vi "user status.vi"(0 "User Index in":i32, 2 "User Info":refnum<vi>, 7 "Userdatabase":path=path "C:/Program Files/National Instruments/LabVIEW 8.2/userdatabase", 9 "User Options":refnum<vi>, 11 "error in (no error)":errorcluster, 12 "User status cmd":T3=enum."Load inputs") -> (3 "valid form":bool, 4 "User Index":i32, 6 "User Information out":T1 {"Country" items=["Afghanistan", "Aland Islands", "Albania", "Algeria", "American Samoa", "Andorra", "Angola", "Anguilla", "Antarctica", "Antigua And Barbuda", "Argentina", "Armenia", "Aruba", "Australia", "Austria", "Azerbaijan", "Bahamas", "Bahrain", "Bangladesh", "Barbados", "Belarus", "Belgium", "Belize", "Benin", "Bermuda", "Bhutan", "Bolivia", "Bosnia And Herzegovina", "Botswana", "Bouvet Island", "Brazil", "British Indian Ocean Territory", "Brunei Darussalam", "Bulgaria", "Burkina Faso", "Burundi", "Cambodia", "Cameroon", "Canada", "Cape Verde", "Cayman Islands", "Central African Republic", "Chad", "Chile", "China", "Christmas Island", "Cocos (Keeling) Islands", "Colombia", "Comoros", "Congo", "Congo, The Democratic Republic Of The", "Cook Islands", "Costa Rica", "Cote D'Ivoire", "Croatia", "Cuba", "Cyprus", "Czech Republic", "Denmark", "Djibouti", "Dominica", "Dominican Republic", "Ecuador", "Egypt", "El Salvador", "Equatorial Guinea", "Eritrea", "Estonia", "Ethiopia", "Falkland Islands (Malvinas)", "Faroe Islands", "Fiji", "Finland", "France", "French Guiana", "French Polynesia", "French Southern Territories", "Gabon", "Gambia", "Georgia", "Germany", "Ghana", "Gibraltar", "Greece", "Greenland", "Grenada", "Guadeloupe", "Guam", "Guatemala", "Guernsey", "Guinea", "Guinea-Bissau", "Guyana", "Haiti", "Heard Island And Mcdonald Islands", "Holy See (Vatican City State)", "Honduras", "Hong Kong", "Hungary", "Iceland", "India", "Indonesia", "Iran, Islamic Republic Of", "Iraq", "Ireland", "Isle Of Man", "Israel", "Italy", "Jamaica", "Japan", "Jersey", "Jordan", "Kazakhstan", "Kenya", "Kiribati", "Korea, Democratic People'S Republic Of", "Korea, Republic Of", "Kuwait", "Kyrgyzstan", "Lao People'S Democratic Republic", "Latvia", "Lebanon", "Lesotho", "Liberia", "Libyan Arab Jamahiriya", "Liechtenstein", "Lithuania", "Luxembourg", "Macao", "Macedonia, The Former Yugoslav Republic Of", "Madagascar", "Malawi", "Malaysia", "Maldives", "Mali", "Malta", "Marshall Islands", "Martinique", "Mauritania", "Mauritius", "Mayotte", "Mexico", "Micronesia, Federated States Of", "Moldova, Republic Of", "Monaco", "Mongolia", "Montserrat", "Morocco", "Mozambique", "Myanmar", "Namibia", "Nauru", "Nepal", "Netherlands", "Netherlands Antilles", "New Caledonia", "New Zealand", "Nicaragua", "Niger", "Nigeria", "Niue", "Norfolk Island", "Northern Mariana Islands", "Norway", "Oman", "Pakistan", "Palau", "Palestinian Territory, Occupied", "Panama", "Papua New Guinea", "Paraguay", "Peru", "Philippines", "Pitcairn", "Poland", "Portugal", "Puerto Rico", "Qatar", "Reunion", "Romania", "Russian Federation", "Rwanda", "Saint Helena", "Saint Kitts And Nevis", "Saint Lucia", "Saint Pierre And Miquelon", "Saint Vincent And The Grenadines", "Samoa", "San Marino", "Sao Tome And Principe", "Saudi Arabia", "Senegal", "Serbia And Montenegro", "Seychelles", "Sierra Leone", "Singapore", "Slovakia", "Slovenia", "Solomon Islands", "Somalia", "South Africa", "South Georgia And The South Sandwich Islands", "Spain", "Sri Lanka", "Sudan", "Suriname", "Svalbard And Jan Mayen", "Swaziland", "Sweden", "Switzerland", "Syrian Arab Republic", "Taiwan, Province Of China", "Tajikistan", "Tanzania, United Republic Of", "Thailand", "Timor-Leste", "Togo", "Tokelau", "Tonga", "Trinidad And Tobago", "Tunisia", "Turkey", "Turkmenistan", "Turks And Caicos Islands", "Tuvalu", "Uganda", "Ukraine", "United Arab Emirates", "United Kingdom", "United States", "United States Minor Outlying Islands", "Uruguay", "Uzbekistan", "Vanuatu", "Venezuela", "Viet Nam", "Virgin Islands, British", "Virgin Islands, U.S.", "Wallis And Futuna", "Western Sahara", "Yemen", "Zambia", "Zimbabwe", "(Not Specified)"]}, 14 "logon status":T4=enum."unregistered email", 15 "error out":errorcluster)   [LabVIEW 2015, in "AguaClara Library.lvlib"]
uses:
  AguaClara Library.lvlib
  language cmd.ctl
  User Information.ctl
  User status.ctl
  User status cmd.ctl
  Country Ring.ctl
panel:
  out "data":T1[](array[typedef]) {"Country" items=["Afghanistan", "Aland Islands", "Albania", "Algeria", "American Samoa", "Andorra", "Angola", "Anguilla", "Antarctica", "Antigua And Barbuda", "Argentina", "Armenia", "Aruba", "Australia", "Austria", "Azerbaijan", "Bahamas", "Bahrain", "Bangladesh", "Barbados", "Belarus", "Belgium", "Belize", "Benin", "Bermuda", "Bhutan", "Bolivia", "Bosnia And Herzegovina", "Botswana", "Bouvet Island", "Brazil", "British Indian Ocean Territory", "Brunei Darussalam", "Bulgaria", "Burkina Faso", "Burundi", "Cambodia", "Cameroon", "Canada", "Cape Verde", "Cayman Islands", "Central African Republic", "Chad", "Chile", "China", "Christmas Island", "Cocos (Keeling) Islands", "Colombia", "Comoros", "Congo", "Congo, The Democratic Republic Of The", "Cook Islands", "Costa Rica", "Cote D'Ivoire", "Croatia", "Cuba", "Cyprus", "Czech Republic", "Denmark", "Djibouti", "Dominica", "Dominican Republic", "Ecuador", "Egypt", "El Salvador", "Equatorial Guinea", "Eritrea", "Estonia", "Ethiopia", "Falkland Islands (Malvinas)", "Faroe Islands", "Fiji", "Finland", "France", "French Guiana", "French Polynesia", "French Southern Territories", "Gabon", "Gambia", "Georgia", "Germany", "Ghana", "Gibraltar", "Greece", "Greenland", "Grenada", "Guadeloupe", "Guam", "Guatemala", "Guernsey", "Guinea", "Guinea-Bissau", "Guyana", "Haiti", "Heard Island And Mcdonald Islands", "Holy See (Vatican City State)", "Honduras", "Hong Kong", "Hungary", "Iceland", "India", "Indonesia", "Iran, Islamic Republic Of", "Iraq", "Ireland", "Isle Of Man", "Israel", "Italy", "Jamaica", "Japan", "Jersey", "Jordan", "Kazakhstan", "Kenya", "Kiribati", "Korea, Democratic People'S Republic Of", "Korea, Republic Of", "Kuwait", "Kyrgyzstan", "Lao People'S Democratic Republic", "Latvia", "Lebanon", "Lesotho", "Liberia", "Libyan Arab Jamahiriya", "Liechtenstein", "Lithuania", "Luxembourg", "Macao", "Macedonia, The Former Yugoslav Republic Of", "Madagascar", "Malawi", "Malaysia", "Maldives", "Mali", "Malta", "Marshall Islands", "Martinique", "Mauritania", "Mauritius", "Mayotte", "Mexico", "Micronesia, Federated States Of", "Moldova, Republic Of", "Monaco", "Mongolia", "Montserrat", "Morocco", "Mozambique", "Myanmar", "Namibia", "Nauru", "Nepal", "Netherlands", "Netherlands Antilles", "New Caledonia", "New Zealand", "Nicaragua", "Niger", "Nigeria", "Niue", "Norfolk Island", "Northern Mariana Islands", "Norway", "Oman", "Pakistan", "Palau", "Palestinian Territory, Occupied", "Panama", "Papua New Guinea", "Paraguay", "Peru", "Philippines", "Pitcairn", "Poland", "Portugal", "Puerto Rico", "Qatar", "Reunion", "Romania", "Russian Federation", "Rwanda", "Saint Helena", "Saint Kitts And Nevis", "Saint Lucia", "Saint Pierre And Miquelon", "Saint Vincent And The Grenadines", "Samoa", "San Marino", "Sao Tome And Principe", "Saudi Arabia", "Senegal", "Serbia And Montenegro", "Seychelles", "Sierra Leone", "Singapore", "Slovakia", "Slovenia", "Solomon Islands", "Somalia", "South Africa", "South Georgia And The South Sandwich Islands", "Spain", "Sri Lanka", "Sudan", "Suriname", "Svalbard And Jan Mayen", "Swaziland", "Sweden", "Switzerland", "Syrian Arab Republic", "Taiwan, Province Of China", "Tajikistan", "Tanzania, United Republic Of", "Thailand", "Timor-Leste", "Togo", "Tokelau", "Tonga", "Trinidad And Tobago", "Tunisia", "Turkey", "Turkmenistan", "Turks And Caicos Islands", "Tuvalu", "Uganda", "Ukraine", "United Arab Emirates", "United Kingdom", "United States", "United States Minor Outlying Islands", "Uruguay", "Uzbekistan", "Vanuatu", "Venezuela", "Viet Nam", "Virgin Islands, British", "Virgin Islands, U.S.", "Wallis And Futuna", "Western Sahara", "Yemen", "Zambia", "Zimbabwe", "(Not Specified)"]}
  out "updated user":bool
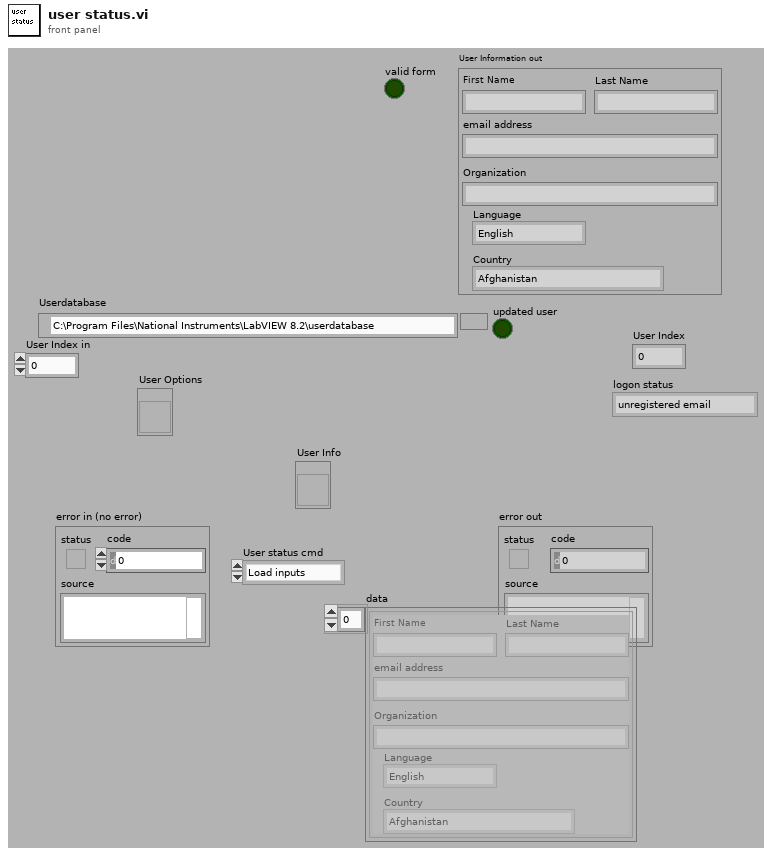
[diagram p1: front panel]
types:
  T1 = typedef "AguaClara Library.lvlib/User Information.ctl" = cluster{"First Name":string, "Last Name":string, "Email Address":string, "Organization":string, "Language":enum16{"English", "Español", "French"}, "Country":T2}
  T2 = typedef "Country Ring.ctl" = u16
  T3 = typedef "AguaClara Library.lvlib/User status cmd.ctl" = enum16{"Load File Path", "Create account", "Update user", "Email password", "Load inputs", "Check status"}
  T4 = typedef "AguaClara Library.lvlib/User status.ctl" = enum16{"invalid email", "unregistered email", "registered email"}
  T5 = enum16{"open", "replace", "create", "open or create", "replace or create", "replace or create with confirmation"}
  T6 = typedef "AguaClara Library.lvlib/language cmd.ctl" = enum16{"load inputs", "choose language", "translate", "load storage variable from file"}
  T7 = cluster{"First Name":string, "Last Name":string, "Email Address":string, "Organization":string, "Language":enum16{"English", "Español", "French"}, "Country":T2}
  T8 = cluster{"First Name":string, "Last Name":string, "Email Address":string, "Organization":string, "Language":enum16{"English", "Español", "French"}, "Country":T2}[]
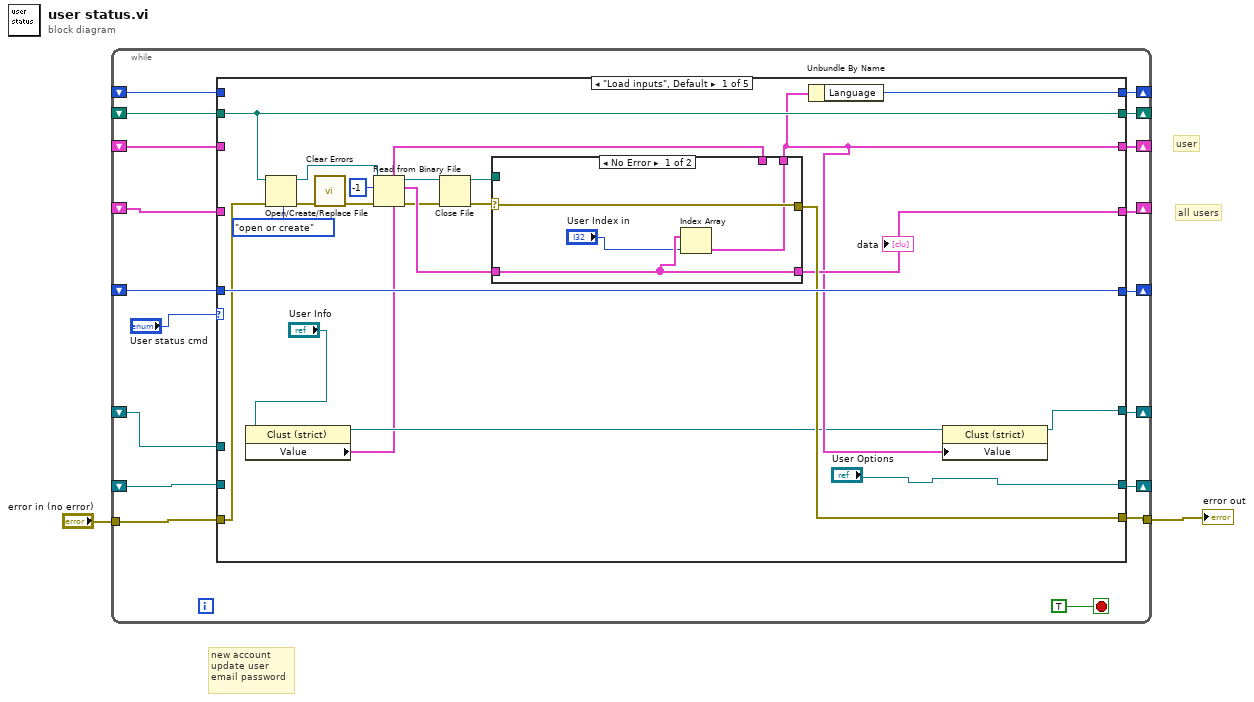
[diagram p0: block diagram]
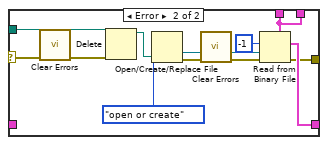
[diagram p2: hidden frame]
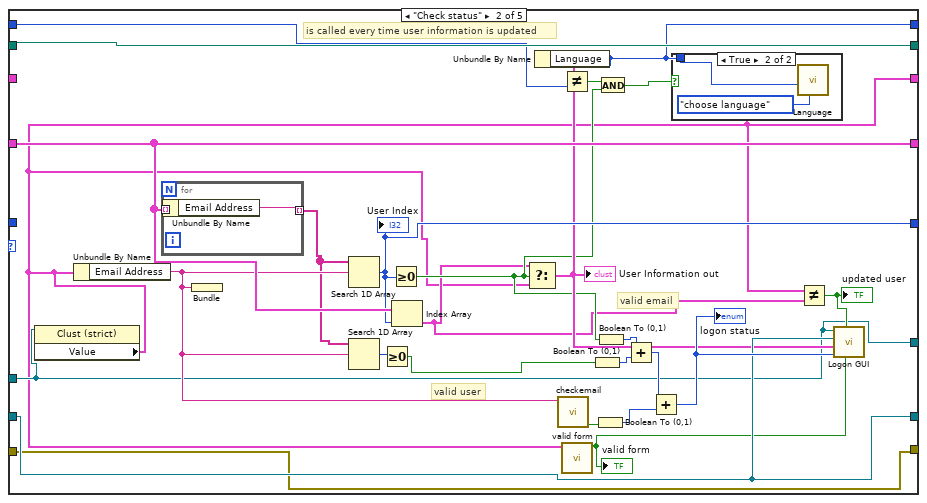
[diagram p3: hidden frame]
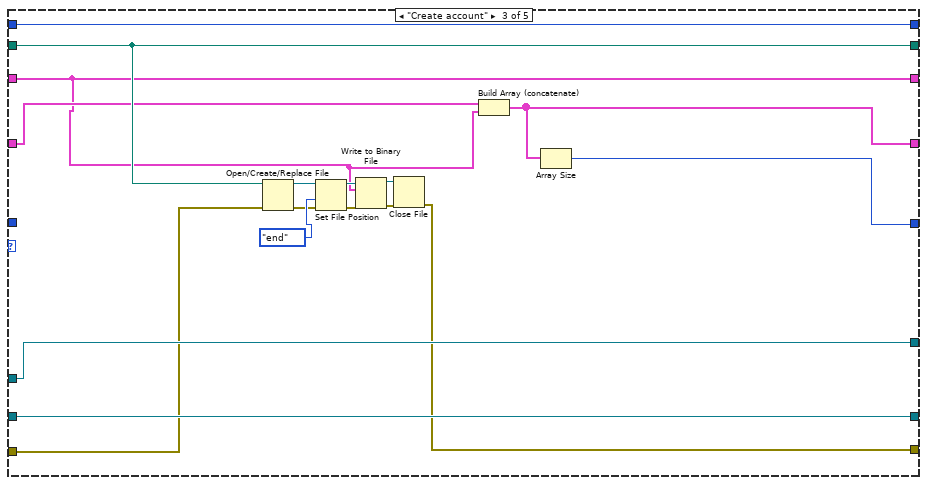
[diagram p5: hidden frame]
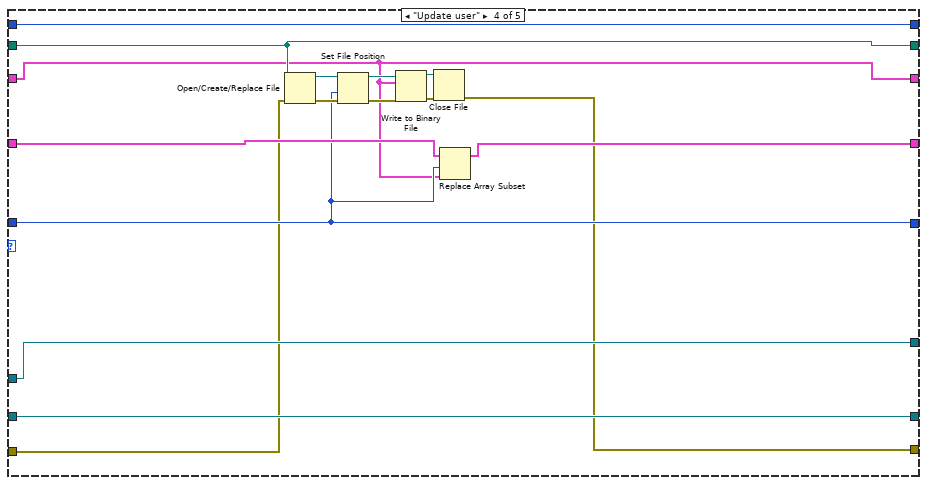
[diagram p6: hidden frame]
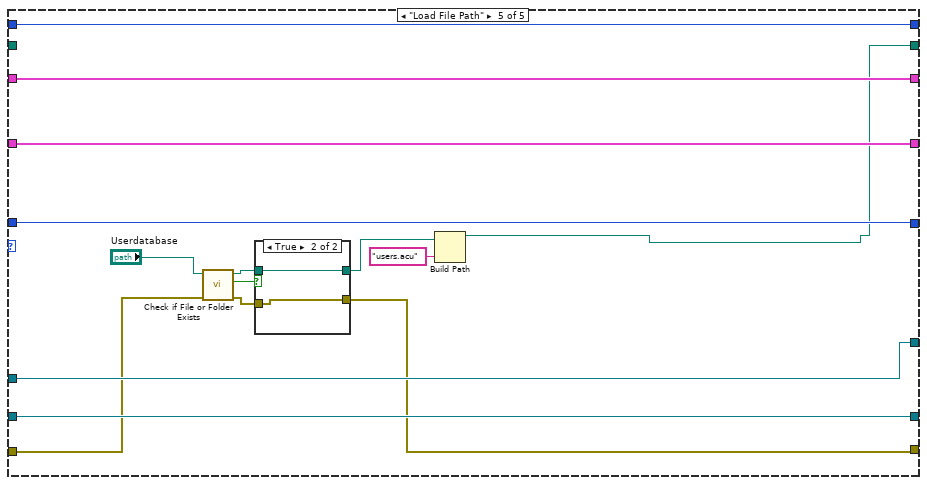
[diagram p7: hidden frame]
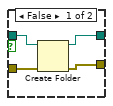
[diagram p8: hidden frame]
diagram:
  # "user"
  # "all users"
  # "new account\nupdate user\nemail password"
  n1 = while {
    shift-right: [w19] -> _
    shift-left: _ -> [w18]
    shift-right: [w17] -> _
    shift-left: _ -> [w16]
    shift-right: [w14] -> _
    shift-left: _ -> [w13]
    shift-right: [w12] -> _
    shift-left: _ -> [w11]
    shift-right: [w10] -> _
    shift-left: _ -> [w9]
    shift-right: [w8] -> _
    shift-left: _ -> [w7]
    tunnel: "error in (no error)" -> [w6]
    tunnel: [w5] -> w1
    shift-right: [w4] -> _
    shift-left: _ -> [w3]
    stop <- TRUE stop-if-true
    n2 = case shown="\"Load inputs\", Default" "User status cmd" {
      tunnel: [w32 w80 w98 w110 w124] -> w19
      tunnel: w18 -> [w32 w80 w98 w110 _]
      tunnel: [w25 w60 w94 w112 w133] -> w17
      tunnel: w16 -> [_ w60 w94 w112 w133]
      tunnel: ["User Options" w74 w93 w111 w132] -> w14
      tunnel: w13 -> [_ w74 w93 w111 w132]
      tunnel: [w26 w76 w96 w113 w135] -> w12
      tunnel: w11 -> [_ w76 w97 w115 w135]
      tunnel: [w38 w73 w95 w114 w134] -> w10
      tunnel: w9 -> [w38 _ _ w114 w134]
      tunnel: [w24 w59 w92 w109 w136] -> w8
      tunnel: w7 -> [_ _ w92 w109 w136]
      tunnel: w6 -> [w37 w70 w91 w108 w125]
      tunnel: [w27 w70 w90 w107 w123] -> w5
      tunnel: [w34 w67 w89 w106 w122] -> w4
      tunnel: w3 -> [_ w69 w89 w106 w122]
      frame "Load inputs", Default {
        n3 = property class="Clust (strict)"(reference="User Info") -> (reference out=w23:refnum<vi>, "Value"=w22:T7)  [unwired: 1 in, 1 out]
        n4 = Open/Create/Replace File(file path (use dialog)=w32, error in=w37, operation (0:open)=T5."open or create") -> (refnum out=w41:refnum<file>, error out=w36:errorcluster)  [unwired: 3 in, 1 out]
        n5 = call <vilib>:"Clear Errors.vi"("error in (no error)"=w36) -> ("error out"=w35:errorcluster)  [unwired: 5 in, 1 out]
        n6 = Read from Binary File(5:w22, 8:w35, 10:-1 ("count"), 11:w41) -> (0:w30:errorcluster, 2:w33:T8, 3:w31:refnum<file>)  [unwired: 2 in, 1 out]
        n7 = Close File(refnum=w31, error in=w30) -> (path=w29:path, error out=w28:errorcluster)
        n8 = case shown="No Error" w28 {
          selector: w28 -> [w46 w49]
          tunnel: w29 -> [_ w53]
          tunnel: [w45 w51] -> w26
          tunnel: w33 -> [w45 _]
          tunnel: w22 -> [_ w47]
          tunnel: [w46 w50] -> w27
          tunnel: [w43 w47] -> w24
          frame No Error {
            n9 = Index Array(array=w45, index="User Index in") -> (element=w43:T7)
          }
          frame Error {
            n10 = call <vilib>:"Clear Errors.vi"("error in (no error)"=w49) -> ("error out"=w48:errorcluster)  [unwired: 5 in, 1 out]
            n11 = Delete(path (use dialog)=w53, error in=w48) -> (deleted path=w52:path)  [unwired: 3 in, 2 out]
            n12 = Open/Create/Replace File(file path (use dialog)=w52, operation (0:open)=T5."open or create") -> (refnum out=w55:refnum<file>, error out=w57:errorcluster)  [unwired: 4 in, 1 out]
            n13 = call <vilib>:"Clear Errors.vi"("error in (no error)"=w57) -> ("error out"=w58:errorcluster)  [unwired: 5 in, 1 out]
            n14 = Read from Binary File(5:w47, 8:w58, 10:-1 ("count"), 11:w55) -> (0:w50:errorcluster, 2:w51:T8)  [unwired: 2 in, 2 out]
          }
        }
        "data" <- w26
        n15 = Unbundle By Name(w24) -> ("Language"=w34:enum16{"English", "Español", "French"})
        n16 = property class="Clust (strict)"(reference=w23, "Value"=w24) -> (reference out=w25:refnum<vi>)  [unwired: 1 in, 1 out]
      }
      frame "Check status" {
        # "is called every time user information is updated"
        # "valid user"
        # "valid email"
        n17 = property class="Clust (strict)"(reference=w60) -> ("Value"=w59:T7)  [unwired: 1 in, 2 out]
        n18 = Unbundle By Name(w59) -> ("Email Address"=w63:string)
        n19 = for {
          tunnel: w76 -> [w88] mode=indexing
          tunnel: [w87] -> w62 mode=indexing
          n20 = Unbundle By Name(w88) -> ("Email Address"=w87:string)
        }
        n21 = Bundle("Email Address"=w63) -> ()  [unwired: 1 in, 1 out]
        n22 = Search 1D Array(1D array=w62, element=w63) -> (index of element=w73:i32)  [unwired: 1 in]
        "User Index" <- w73
        n23 = Search 1D Array(1D array=w62, element=w63) -> (index of element=w84:i32)  [unwired: 1 in]
        n24 = Greater Or Equal To 0?(x=w84) -> (x >= 0?=w83:bool)
        n25 = Greater Or Equal To 0?(x=w73) -> (x >= 0?=w64:bool)
        n26 = Index Array(array=w76, index=w73) -> (element=w61:T7)
        n27 = Select(t=w61, s=w64, f=w59) -> (s? t:f=w68:T7)
        "User Information out" <- w68
        n28 = Unbundle By Name(w68) -> ("Language"=w67:enum16{"English", "Español", "French"})
        n29 = call "checkemail.vi"("email"=w63) -> ("valid email"=w79:bool)  [unwired: 7 in, 3 out]
        n30 = Not Equal?(x=w67, y=w69) -> (x != y?=w66:bool)
        n31 = call "valid form.vi"("User Information"=w59) -> ("valid form"=w71:bool)  [unwired: 10 in]
        "valid form" <- w71
        n32 = Boolean To (0,1)(Boolean=w83) -> (0, 1=w81:i16)
        n33 = Boolean To (0,1)(Boolean=w79) -> (0, 1=w78:i16)
        n34 = Boolean To (0,1)(Boolean=w64) -> (0, 1=w82:i16)
        n35 = And(x=w66, y=w64) -> (x .and. y?=w65:bool)
        n36 = Add(x=w82, y=w81) -> (x+y=w77:i16)
        n37 = Add(x=w77, y=w78) -> (x+y=w75:i16)
        "logon status" <- w75
        n38 = case shown="True" w65 {
          tunnel: w67 -> [_ w85]
          frame False {
          }
          frame True {
            n39 = call "Language.vi"("language cmd"=language_cmd."choose language", "Language"=w85) -> ()  [unwired: 8 in, 2 out]
          }
        }
        n40 = Not Equal?(x=w59, y=w61) -> (x != y?=w72:bool)
        "updated user" <- w72
        n41 = call "Logon GUI.vi"("updated user"=w72, "valid form"=w71, "logon status"=w75, "User Information from db"=w68, "User Options"=w74, "User Info"=w60) -> ()  [unwired: 6 in]
      }
      frame "Create account" {
        n42 = Open/Create/Replace File(file path (use dialog)=w98, error in=w91) -> (refnum out=w102:refnum<file>, error out=w99:errorcluster)  [unwired: 4 in, 1 out]
        n43 = Set File Position(refnum=w102, from (0:start)=enum16{"start", "end", "current"}."end", error in=w99) -> (refnum out=w101:refnum<file>, error out=w100:errorcluster)  [unwired: 1 in]
        n44 = Write to Binary File(file (use dialog)=w101, data=w92, error in=w100) -> (refnum out=w103:refnum<file>, error out=w104:errorcluster)  [unwired: 3 in, 1 out]
        n45 = Close File(refnum=w103, error in=w104) -> (error out=w90:errorcluster)  [unwired: 1 out]
        n46 = Build Array (concatenate)(w97, w92) -> (w96:T8)
        n47 = Array Size(array=w96) -> (size(s)=w95:i32)
      }
      frame "Update user" {
        n48 = Open/Create/Replace File(file path (use dialog)=w110, error in=w108) -> (refnum out=w121:refnum<file>, error out=w118:errorcluster)  [unwired: 4 in, 1 out]
        n49 = Set File Position(refnum=w121, from (0:start)=w114, error in=w118) -> (refnum out=w120:refnum<file>, error out=w117:errorcluster)  [unwired: 1 in]
        n50 = Write to Binary File(file (use dialog)=w120, data=w109, error in=w117) -> (refnum out=w119:refnum<file>, error out=w116:errorcluster)  [unwired: 3 in, 1 out]
        n51 = Close File(refnum=w119, error in=w116) -> (error out=w107:errorcluster)  [unwired: 1 out]
        n52 = Replace Array Subset(array=w115, new element=w109, index=w114) -> (w113:T8)
      }
      frame "Load File Path" {
        n53 = call <vilib>:"Check if File or Folder Exists.vi"("error in (no error)"=w125, "path"="Userdatabase") -> ("error out"=w127:errorcluster, "file or folder exists?"=w129:bool, "dup path"=w130:path)  [unwired: 7 in]
        n54 = case shown="True" w129 {
          tunnel: w130 -> [w140 w142]
          tunnel: [w139 w142] -> w126
          tunnel: w127 -> [w138 w141]
          tunnel: [w137 w141] -> w123
          frame False {
            n55 = Create Folder(path (use dialog)=w140, error in=w138) -> (created path=w139:path, error out=w137:errorcluster)  [unwired: 1 in, 1 out]
          }
          frame True {
          }
        }
        n56 = Build Path(base path=w126, name or relative path="users.acu") -> (appended path=w124:path)
      }
    }
  }
  "error out" <- w1
